vi "Before.vi"(8 "Error In":errorcluster, 11 "Session In":refnum<class "Session.lvclass">) -> (0 "Error Out":errorcluster, 1 "Remote Link Path":string, 2 "Remote Source Path":string, 3 "SFTP Out":refnum<class "SFTP.lvclass">)   [LabVIEW 2018, in "Tests.lvlib" / "SFTP.lvlib"]
uses:
  SFTP.lvlib
  src/Toolkit/SFTP/SFTP.lvclass
  src/Toolkit/Session/Session.lvclass
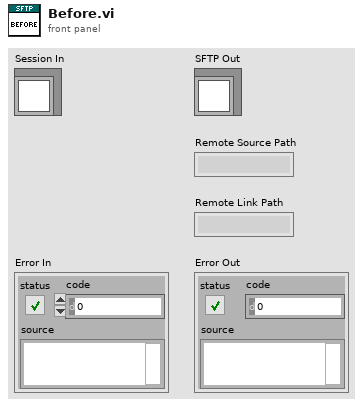
[diagram p1: front panel]
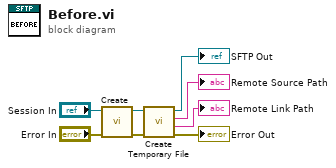
[diagram p0: block diagram]
diagram:
  n1 = call "Create.vi"("Error In"="Error In", "Session"="Session In") -> ("Error Out"=w3:errorcluster, "SFTP"=w4:refnum<class "SFTP.lvclass">)  [unwired: 8 in]
  n2 = call "Create Temporary File.vi"("Error In"=w3, "SFTP In"=w4) -> ("Error Out"=→"Error Out":errorcluster, "Remote Link Path"=→"Remote Link Path":string, "Remote Source Path"=→"Remote Source Path":string, "SFTP Out"=→"SFTP Out":refnum<class "SFTP.lvclass">)  [unwired: 6 in]
